vi "Température to puissance.vi"(10 "Longueur d'onde":dbl, 11 "Température max":dbl) -> (3 "Puissance":dbl)   [LabVIEW 2018]
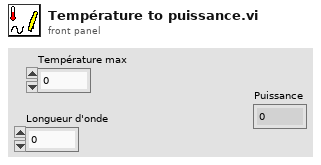
[diagram p1: front panel]
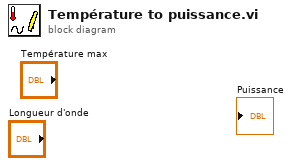
[diagram p0: block diagram]
diagram:
